vi "Keithley DMM6500 DAQ6500 Series Scanning Resistors 4wire Measurements.vi"() -> ()   [LabVIEW 2023]
doc: "This example shows how to do 4-wire resistance measurement."
uses:
  <instrlib>/Keithley DMM6500 DAQ6500 Series/Public/Data/Read (Multiple Points).vi
  <instrlib>/Keithley DMM6500 DAQ6500 Series/Keithley DMM6500 DAQ6500 Series.lvlib
panel:
  in  "Buffer Element2 ()":i32(ring) items=["", "Date", "Extra", "Formatted", "Fractional", "Reading", "Relative", "Seconds", "Status", "Time", "Tstamp", "Unit", "CHAN", "Extra Form", "Extra Unit"]
  in  "Buffer Element1 ()":i32(ring) items=["", "Date", "Extra", "Formatted", "Fractional", "Reading", "Relative", "Seconds", "Status", "Time", "Tstamp", "Unit", "CHAN", "Extra Format", "Extra Unit"]
  in  "Channel List 3 (\"105,106\")":string="105,106"
  in  "Auto Range 3 (F: Disable)":bool
  in  "Manual Range 3 (1)":dbl=1.0
  in  "Channel List 2 (\"103,104\")":string="103,104"
  in  "Auto Range 2 (F: Disable)":bool
  in  "Manual Range 2 (10)":dbl=10.0
  in  "Channel List 1 (\"101,102\")":string="101,102"
  out "Measurements":dbl[](array[numeric])
  in  "Auto Range 1 (F: Disable)":bool
  in  "Delay Seconds (60 s)":dbl=60.0
  in  "Manual Range 1 (100)":dbl=100.0
  in  "Scan Count (100)":u32=100
  in  "Buffer Size (600)":u32=600
  in  "Buffer Name (defbuffer1)":string="defbuffer1"
  in  "Channel List (\"101:106\")":string="101:106"
  in  "VISA resource name":refnum<visa-resource-name>
  # "(c) 2018-2022 National Instruments.  ALL RIGHTS RESERVED."
  # "The combination of channel list in \"Channel List 1\", \"Channel List 2\" and \"Channel List 3\" should be equal to control \"Channel List\""
  # "This example application demonstrates how to use the DAQ6500 Series to accurately measure resistance across multiple devices. To obtain the best results, the 4-wire (Kelvin) measurement method and offset compensation are used for this test."
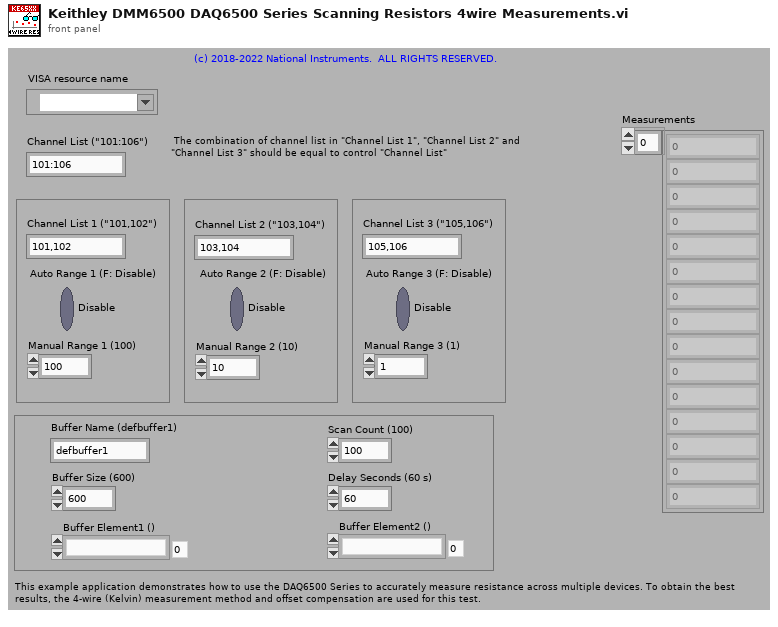
[diagram p1: front panel]
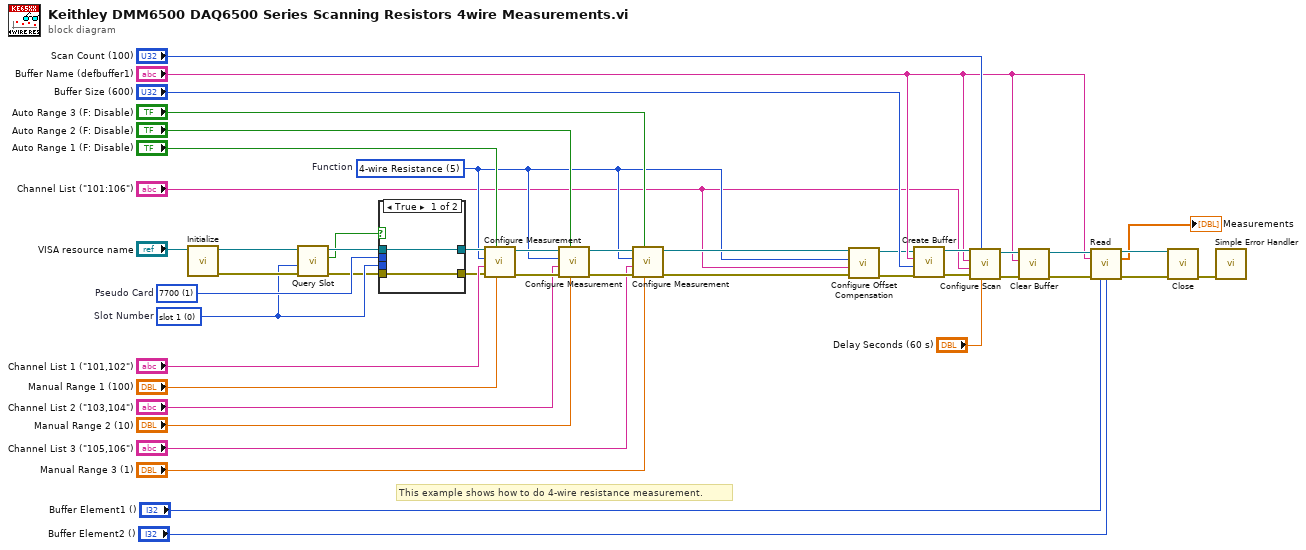
[diagram p0: block diagram]
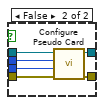
[diagram p2: hidden frame]
diagram:
  w5 = 0 items=["slot 1", "slot 2"]  # Slot Number
  w30 = 1 items=["0", "7700", "7701", "7702", "7703", "7705", "7706", "7707", "7708", "7709", "7710", "7711", "7712"]  # Pseudo Card
  w9 = 5 items=[" Voltage DC", "Voltage AC", "Current DC", "Current AC", "Resistance", "4-wire Resistance", "Diode", "Capacitance", "Temperature", "Continuity", "Frequency", "Period", "Voltage Ratio", "Digitize Voltage", "Digitize Current"]  # Function
  # "This example shows how to do 4-wire resistance measurement."
  n1 = call <instrlib>:"Initialize.vi"("VISA resource name"="VISA resource name") -> ("error out"=w6:errorcluster, "VISA resource name out"=w43:refnum<visa-resource-name>)  [unwired: 9 in]
  n2 = call <instrlib>:"Query Slot.vi"("error in (no error)"=w6, "Slot Number(0: slot 1)"=w5, "VISA resource name"=w43) -> ("error out"=w4:errorcluster, "Real Card In Slot"=w3:bool, "VISA resource name out"=w7:refnum<visa-resource-name>)  [unwired: 6 in]
  n3 = case shown="True" w3 {
    tunnel: w30 -> [_ w53]
    tunnel: [w47 w52] -> w15
    tunnel: [w46 w51] -> w14
    tunnel: w7 -> [w47 w50]
    tunnel: w5 -> [_ w49]
    tunnel: w4 -> [w46 w48]
    frame True {
    }
    frame False {
      n4 = call <instrlib>:"Configure Pseudo Card.vi"("error in (no error)"=w48, "Slot Number (0: slot1)"=w49, "Pseudo Card (0:No pseudocard)"=w53, "VISA resource name"=w50) -> ("error out"=w51:errorcluster, "VISA resource name out"=w52:refnum<visa-resource-name>)  [unwired: 6 in]
    }
  }
  n5 = call <instrlib>:"Configure Measurement.vi"("Manual Range (1)"="Manual Range 1 (100)", "Auto Range (T: Enable)"="Auto Range 1 (F: Disable)", "error in (no error)"=w14, "Channel List(\"\")"="Channel List 1 (\"101,102\")", "Function (0: Voltage DC)"=w9, "VISA resource name"=w15) -> ("error out"=w24:errorcluster, "VISA resource name out"=w25:refnum<visa-resource-name>)  [unwired: 4 in]
  n6 = call <instrlib>:"Configure Measurement.vi"("Manual Range (1)"="Manual Range 2 (10)", "Auto Range (T: Enable)"="Auto Range 2 (F: Disable)", "error in (no error)"=w24, "Channel List(\"\")"="Channel List 2 (\"103,104\")", "Function (0: Voltage DC)"=w9, "VISA resource name"=w25) -> ("error out"=w22:errorcluster, "VISA resource name out"=w23:refnum<visa-resource-name>)  [unwired: 4 in]
  n7 = call <instrlib>:"Configure Measurement.vi"("Manual Range (1)"="Manual Range 3 (1)", "Auto Range (T: Enable)"="Auto Range 3 (F: Disable)", "error in (no error)"=w22, "Channel List(\"\")"="Channel List 3 (\"105,106\")", "Function (0: Voltage DC)"=w9, "VISA resource name"=w23) -> ("error out"=w12:errorcluster, "VISA resource name out"=w13:refnum<visa-resource-name>)  [unwired: 4 in]
  n8 = call <instrlib>:"Configure Offset Compensation.vi"("error in (no error)"=w12, "Channel List(\"\")"="Channel List (\"101:106\")", "Function (5: 4-wire resistance)"=w9, "VISA resource name"=w13) -> ("error out"=w11:errorcluster, "VISA resource name out"=w10:refnum<visa-resource-name>)  [unwired: 6 in]
  n9 = call <instrlib>:"Create Buffer.vi"("error in (no error)"=w11, "Buffer Size (10)"="Buffer Size (600)", "Buffer Name (\"\")"="Buffer Name (defbuffer1)", "VISA resource name"=w10) -> ("error out"=w37:errorcluster, "VISA resource name out"=w38:refnum<visa-resource-name>)  [unwired: 6 in]
  n10 = call <instrlib>:"Configure Scan.vi"("Delay Seconds (0 s)"="Delay Seconds (60 s)", "Scan Count (1)"="Scan Count (100)", "error in (no error)"=w37, "Channel List(\"\")"="Channel List (\"101:106\")", "Reading Buffer (\"\")"="Buffer Name (defbuffer1)", "VISA resource name"=w38) -> ("error out"=w40:errorcluster, "VISA resource name out"=w39:refnum<visa-resource-name>)  [unwired: 4 in]
  n11 = call <instrlib>:"Clear Buffer.vi"("error in (no error)"=w40, "Buffer Name (\"\")"="Buffer Name (defbuffer1)", "VISA resource name"=w39) -> ("error out"=w34:errorcluster, "VISA resource name out"=w35:refnum<visa-resource-name>)  [unwired: 7 in]
  n12 = call-poly <instrlib>:"Read.vi"("VISA resource name"=w35, "Buffer Name (\"\")"="Buffer Name (defbuffer1)", "error in (no error)"=w34, "Buffer Element1 ()"="Buffer Element1 ()", "Buffer Element2 ()"="Buffer Element2 ()") -> ("VISA resource name out"=w32:refnum<visa-resource-name>, "Measurements"=→"Measurements":dbl[], "error out"=w33:errorcluster)  [unwired: 8 in]
  n13 = call <instrlib>:"Close.vi"("error in (no error)"=w33, "VISA resource name"=w32) -> ("error out"=w45:errorcluster)  [unwired: 9 in]
  n14 = call <vilib>:"Simple Error Handler.vi"("error in (no error)"=w45) -> ()  [unwired: 4 in, 5 out]
